vi "LJUD_DoubleToStringAddress.vi"(8 "error in":errorcluster, 10 "HexDot":bool, 11 "Double":dbl format="%.2f") -> (0 "error out":errorcluster, 3 "String":string="192.168.1.209")   [LabVIEW 2021]
doc: "Some special-channels of the config IOType pass IP\naddress (and others) in a double. This function is used\nto convert the double into a string in normal decimal-dot\nor hex-dot notation.\n\nDocumented in Section 4.2 of the device's datasheet."
uses:
  labjackud.dll
panel:
  # "Some special-channels of the config IOType pass IP\naddress (and others) in a double. This function is used\nto convert the double into a string in normal decimal-dot\nor hex-dot notation.\n\nDocumented in Section 4.2 of the device's datasheet."
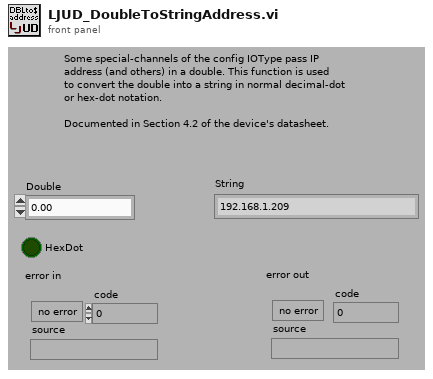
[diagram p1: front panel]
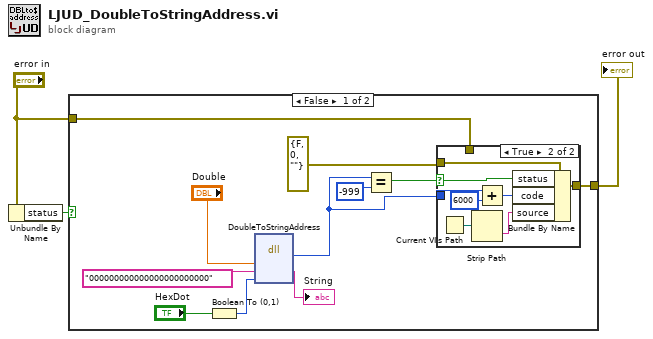
[diagram p0: block diagram]
diagram:
  n1 = Unbundle By Name("error in") -> ("status"=w1:bool)
  n2 = case shown="False" w1 {
    tunnel: [w13 w24] -> w3
    tunnel: "error in" -> [w4 w24]
    frame False {
      n3 = Boolean To (0,1)(Boolean="HexDot") -> (0, 1=w8:i16)
      n4 = dll-call lib="labjackud.dll" fn="DoubleToStringAddress"("Number"="Double", "String"="000000000000000000000000", "HexDot"=w8) -> (w10:i32, "String"=→"String":string)  [unwired: 5 in, 2 out]
      n5 = Equal?(x=w10, y=-999) -> (x = y?=w11:bool)
      n6 = case shown="True" w11 {
        selector: w11 -> [_ w22]
        tunnel: [w15 w23] -> w13
        tunnel: errorcluster {"status"=FALSE, "code"=0, "source"=""} ("error IO") -> [_ w21]
        tunnel: w10 -> [_ w17]
        tunnel: w4 -> [w15 _]
        frame False {
        }
        frame True {
          n7 = Current VI's Path() -> (path=w19:path)
          n8 = Strip Path(path=w19) -> (name=w20:string)  [unwired: 1 out]
          n9 = Add(x=w17, y=6000) -> (x+y=w18:i32)
          n10 = Bundle By Name(cluster=w21, "status"=w22, "code"=w18, "source"=w20) -> (w23:errorcluster)
        }
      }
    }
    frame True {
    }
  }
  "error out" <- w3
